vi "get_data_from_server.vi"(8 "error in (no error)":errorcluster, 11 "TCP Network Connection in":refnum<k5>) -> (0 "error out":errorcluster, 2 "connection ID out":refnum<k5>, 3 "input cluster":T1)   [LabVIEW 2020]
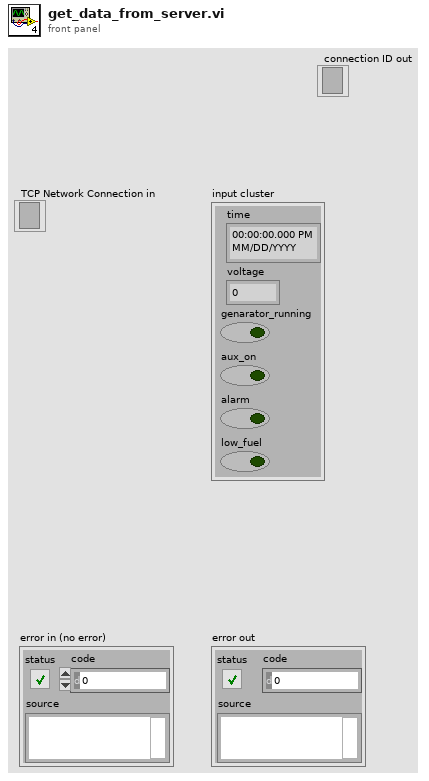
[diagram p1: front panel]
types:
  T1 = cluster{"time":timestamp, "voltage":dbl, "genarator_running":bool, "aux_on":bool, "alarm":bool, "low_fuel":bool}
  T2 = cluster{"byteorder":string, "content-type":string, "content-encoding":string, "content-length":i32}
  T3 = enum16{"Standard", "Buffered", "CRLF", "Immediate"}
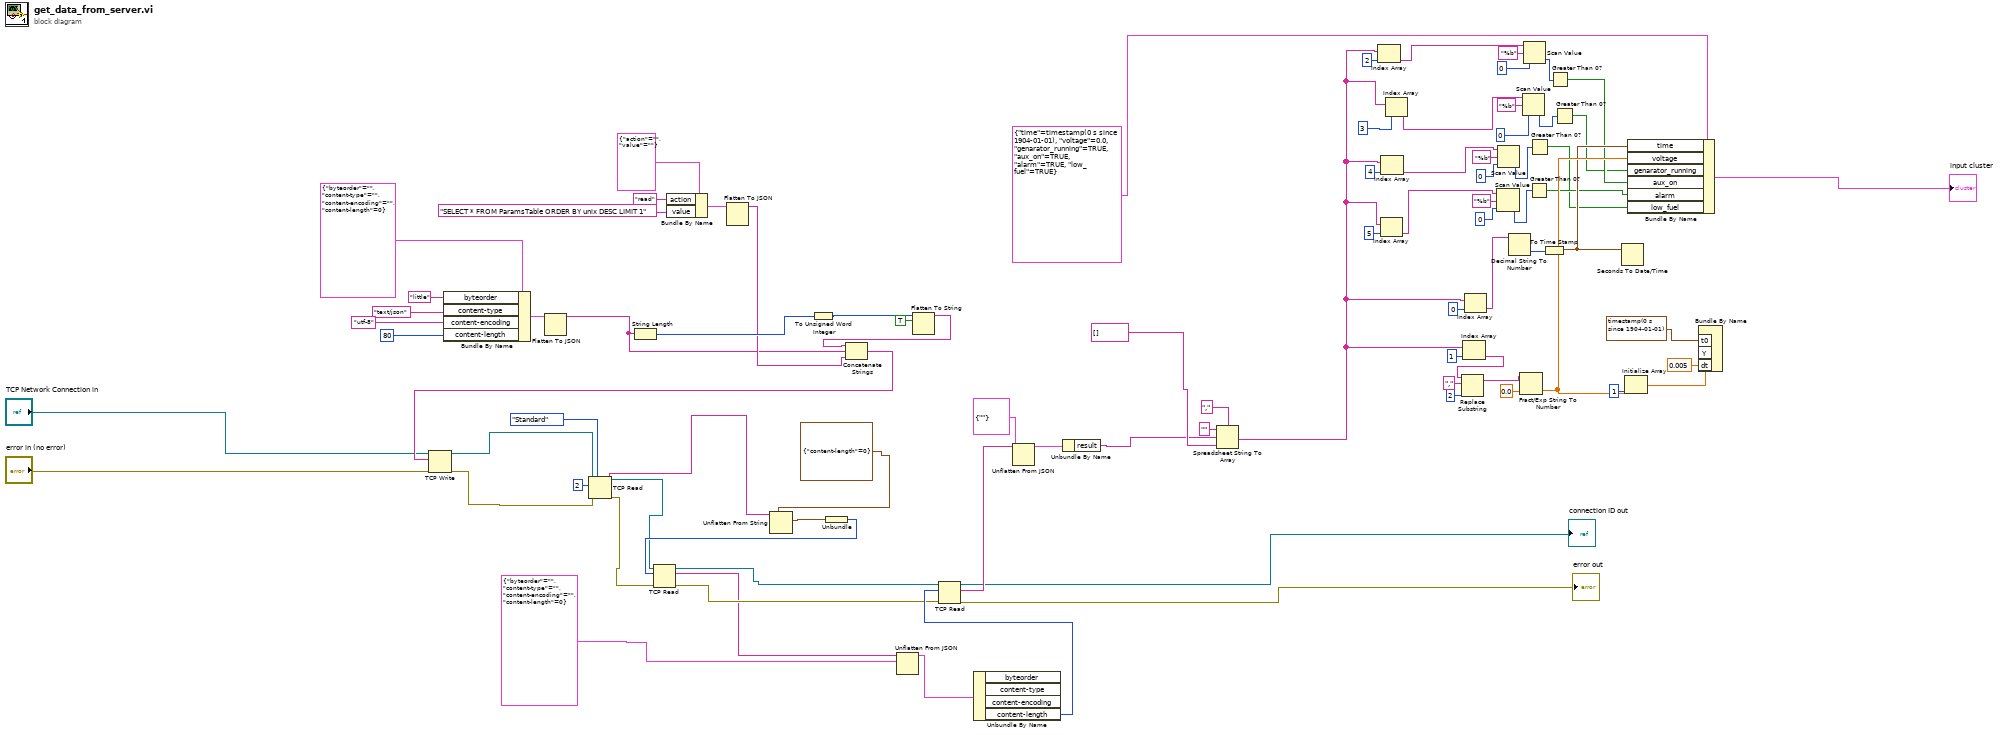
[diagram p0: block diagram]
diagram:
  n1 = Bundle By Name(cluster=T2 {"byteorder"="", "content-type"="", "content-encoding"="", "content-length"=0} ("input cluster"), "byteorder"="little", "content-type"="text/json" ("content_type"), "content-encoding"="utf-8", "content-length"=80) -> (w14:T2)
  n2 = Flatten To JSON(anything=w14) -> (JSON string=w21:string)  [unwired: 2 in, 1 out]
  n3 = String Length(string=w21) -> (length=w26:i32)
  n4 = Bundle By Name(cluster=cluster{"action":string, "value":string} {"action"="", "value"=""} ("input cluster"), "action"="read" ("byteorder"), "value"="SELECT * FROM ParamsTable ORDER BY unix DESC LIMIT 1" ("content_type")) -> (w20:cluster{"action":string, "value":string})
  n5 = Flatten To JSON(anything=w20) -> (JSON string=w22:string)  [unwired: 2 in, 1 out]
  n6 = To Unsigned Word Integer(number=w26) -> (unsigned 16bit integer=w27:u16)
  n7 = Flatten To String(anything=w27, prepend array or string size? (T)=TRUE) -> (data string=w24:string)  [unwired: 2 in, 2 out]
  n8 = Concatenate Strings(w24, w21, w22) -> (w23:string)
  n9 = TCP Write(connection ID="TCP Network Connection in", data in=w23, error in (no error)="error in (no error)") -> (connection ID out=w9:refnum<k5>, error out=w36:errorcluster)  [unwired: 1 in, 1 out]
  n10 = TCP Read(connection ID=w9, bytes to read=2, error in (no error)=w36, 7:T3."Standard" ("mode (standard)")) -> (connection ID out=w33:refnum<k5>, data out=w29:string, error out=w32:errorcluster)  [unwired: 1 in]
  n11 = Unflatten From String(type=cluster{"content-length":u16} {"content-length"=0}, binary string=w29) -> (value=w31:cluster{"content-length":u16})  [unwired: 3 in, 2 out]
  n12 = Unbundle(w31) -> ("content-length"=w44:u16)
  n13 = TCP Read(connection ID=w33, bytes to read=w44, error in (no error)=w32) -> (connection ID out=w40:refnum<k5>, data out=w34:string, error out=w38:errorcluster)  [unwired: 2 in]
  n14 = Unflatten From JSON(JSON string=w34, type and defaults=T2 {"byteorder"="", "content-type"="", "content-encoding"="", "content-length"=0} ("input cluster")) -> (value=w37:T2)  [unwired: 5 in, 1 out]
  n15 = Unbundle By Name(w37) -> ("content-length"=w39:i32)  [unwired: 3 out]
  n16 = TCP Read(connection ID=w40, bytes to read=w39, error in (no error)=w38) -> (connection ID out=→"connection ID out":refnum<k5>, data out=w41:string, error out=→"error out":errorcluster)  [unwired: 2 in]
  n17 = Unflatten From JSON(JSON string=w41, type and defaults=cluster{"result":string} {"result"=""}) -> (value=w42:cluster{"result":string})  [unwired: 5 in, 1 out]
  n18 = Unbundle By Name(w42) -> ("result"=w47:string)
  n19 = Spreadsheet String To Array(delimiter (Tab)=",", format string="", spreadsheet string=w47, array type (2D Dbl)=string[] []) -> (array=w68:string[])
  n20 = Index Array(array=w68, index=2) -> (element=w69:string)
  n21 = Index Array(array=w68, index=5) -> (element=w84:string)
  n22 = Index Array(array=w68, index=4) -> (element=w80:string)
  n23 = Index Array(array=w68, index=3) -> (element=w76:string)
  n24 = Index Array(array=w68, index=1) -> (element=w58:string)
  n25 = Replace Substring(3:2 ("offset (0)"), 4:"," ("substring (\"\")"), 5:w58) -> (1:w61:string)  [unwired: 1 in, 1 out]
  n26 = Index Array(array=w68, index=0) -> (element=w52:string)
  n27 = Scan Value(string=w84, format string="%b", default (0 dbl)=u8 0) -> (value=w81:u8)  [unwired: 1 out]
  n28 = Scan Value(string=w80, format string="%b", default (0 dbl)=u8 0) -> (value=w77:u8)  [unwired: 1 out]
  n29 = Decimal String To Number(string=w52) -> (number=w51:i32)  [unwired: 2 in, 1 out]
  n30 = Fract/Exp String To Number(string=w61, default (0 dbl)=0.0 ("default (0 I32)")) -> (number=w63:dbl)  [unwired: 2 in, 1 out]
  n31 = Scan Value(string=w76, format string="%b", default (0 dbl)=u8 0) -> (value=w75:u8)  [unwired: 1 out]
  n32 = Scan Value(string=w69, format string="%b", default (0 dbl)=u8 0) -> (value=w72:u8)  [unwired: 1 out]
  n33 = Greater Than 0?(x=w81) -> (x > 0?=w2:bool)
  n34 = Greater Than 0?(x=w77) -> (x > 0?=w1:bool)
  n35 = To Time Stamp(1:w51) -> (0:w62:timestamp)
  n36 = Greater Than 0?(x=w72) -> (x > 0?=w4:bool)
  n37 = Greater Than 0?(x=w75) -> (x > 0?=w3:bool)
  n38 = Seconds To Date/Time(time stamp (now)=w62) -> ()  [unwired: 1 in, 1 out]
  n39 = Initialize Array(w63, 1 ("dimension size")) -> (w57:dbl[])
  n40 = Bundle By Name(cluster=T1 {"time"=timestamp(0 s since 1904-01-01), "voltage"=0.0, "genarator_running"=TRUE, "aux_on"=TRUE, "alarm"=TRUE, "low_fuel"=TRUE} ("input cluster"), "time"=w62, "voltage"=w63, "genarator_running"=w3, "aux_on"=w4, "alarm"=w2, "low_fuel"=w1) -> (→"input cluster":T1)
  n41 = Bundle By Name("t0"=timestamp(0 s since 1904-01-01), "Y"=w57, "dt"=0.005) -> ()  [unwired: 1 in, 1 out]
